vi "_FPGA_Accumulator_U32.vi"(6 "Clk_in":bool, 7 "Reset_latch":bool, 8 "U32_shift_in":u32, 10 "U32_in":u32, 11 "Decrease / increase":bool=TRUE) -> (2 "Accumulated_U32_out":u32)   [LabVIEW 2018]
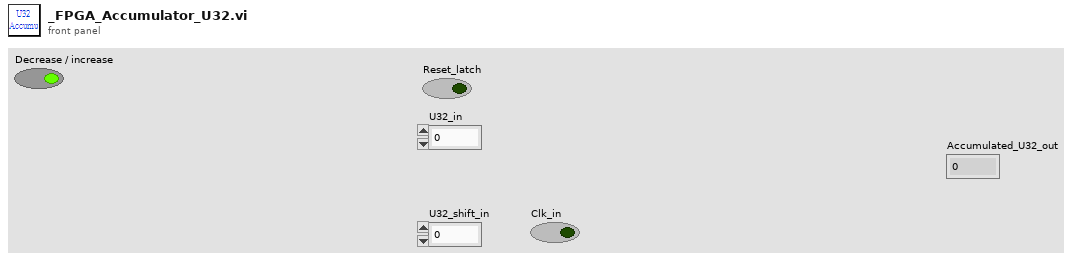
[diagram p1: front panel]
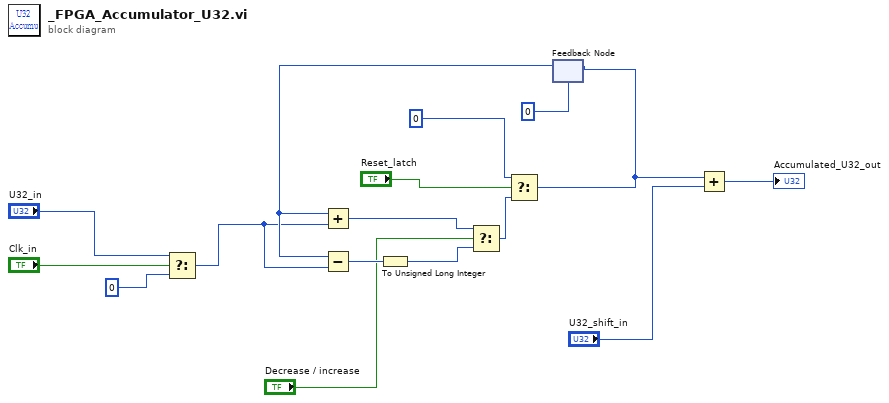
[diagram p0: block diagram]
diagram:
  n1 = Select(t="U32_in", s="Clk_in", f=u32 0) -> (s? t:f=w6:u32)
  n2 = feedback #1(u32 0 ("t")) -> (w7:u32)
  n3 = Add(x=w7, y=w6) -> (x+y=w4:u32)
  n4 = Subtract(x=w7, y=w6) -> (x-y=w5:u32)
  n5 = To Unsigned Long Integer(number=w5) -> (unsigned 32bit integer=w3:u32)
  n6 = Select(t=w4, s="Decrease / increase", f=w3) -> (s? t:f=w2:u32)
  n7 = Select(t=u32 0, s="Reset_latch", f=w2) -> (s? t:f=w8:u32)
  n8 = feedback-in #1(w8) -> ()
  n9 = Add(x=w8, y="U32_shift_in") -> (x+y=→"Accumulated_U32_out":u32)
